vi "Read Channel Names.vi"(8 "error in (no error)":errorcluster, 11 "Node Ptr":T1 format="%.0x") -> (0 "error out":errorcluster, 2 "Channel Names":string[](array[string]), 3 "Node Ptr out":T1 format="%.0x")   [LabVIEW 2016, in "UDP-Custom-Device System Explorer.lvlib"]
uses:
  UDP-Custom-Device System Explorer.lvlib
  <vilib>/NI Veristand/Custom Device API/Custom Device Item Ref.ctl
  Shared/Constants.vi
  <vilib>/NI Veristand/Custom Device API/Get Item Property (String Array).vi
  <vilib>/NI VeriStand/Custom Device API/Custom Device API.lvlib
  Shared/UDP-Custom-Device Shared.lvlib
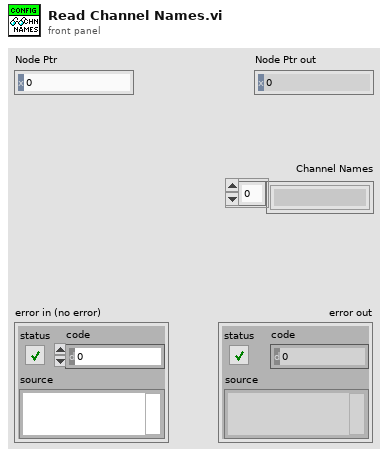
[diagram p1: front panel]
types:
  T1 = typedef "Custom Device API.lvlib/Custom Device Item Ref.ctl" = u64
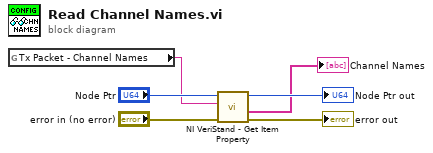
[diagram p0: block diagram]
diagram:
  n1 = global read "Constants.vi" "Tx Packet - Channel Names"() -> (w2:string)
  n2 = call-poly <vilib>:"NI VeriStand - Get Item Property.vi"("error in (no error)"="error in (no error)", "Property Name"=w2, "Item Ref in"="Node Ptr") -> ("error out"=→"error out":errorcluster, "Value"=→"Channel Names":string[], "Item Ref out"=→"Node Ptr out":T1)  [unwired: 5 in, 1 out]
